vi "IV_Fast.vi"(8 "error in":errorcluster, 11 "Transport":refnum<class "Transport.lvclass">) -> (0 "error out":errorcluster, 3 "Transport out":refnum<class "Transport.lvclass">)   [LabVIEW 2016, in "Transport.lvclass"]
uses:
  Transport.lvclass
  Control Experiment/Typedefs/Instruments--cluster.ctl
  <userlib>/LevyLab/Krohn Hite 7008/Instrument.KH7008.lvclass
  <userlib>/LevyLab/Lockin-Multichannel/Instrument.Lockin/Instrument.Lockin.lvclass
  <userlib>/LevyLab/Levylab Instruments/Instrument Types/Cryostat/Instrument.Cryostat.lvclass
  <userlib>/LevyLab/Levylab Instruments/Instrument Types/CBridge/Instrument.CBridge.lvclass
  <userlib>/LevyLab/Levylab Instruments/Instrument Types/Optical Delay Line/Instrument.OpticalDelayLine.lvclass
  <userlib>/LevyLab/Levylab Instruments/Instrument Types/Strain/Instrument.Strain.lvclass
  <userlib>/LevyLab/Levylab Instruments/Instrument Types/VNA/Instrument.VNA.lvclass
  <userlib>/LevyLab/Levylab Instruments/Instrument Types/VSource/Instrument.VSource.lvclass
  <userlib>/LevyLab/Lockin-Multichannel/LockinDAQ/Typedefs/AO-cluster.ctl
  <userlib>/LevyLab/Lockin-Multichannel/LockinDAQ/Typedefs/Function-enum.ctl
  Transport.lvclass/Transport.ctl
  Control Experiment/Control Experiment.lvclass/Control Experiment.ctl
  Control Experiment/Control Experiment.lvclass
  <userlib>/LevyLab/Lockin-Multichannel/LockinDAQ/LockinDAQ.lvclass
panel:
  in  "OK":bool
  out "4Term":cluster{dbl[], dbl[]}[](graph)
  out "2Term":T1(graph)
  in  "Tab Control":T2(tab)
  in  "decimating factor":i32=1
  in  "low cutoff freq: fl":dbl=0.01 format="%0.4f"
  out "Temp":dbl
  in  "offset":dbl[](array[numeric])=[0.0, 0.0, 0.0, 0.0, 0.0, 0.0, 0.0, 0.0] format="%_6p"
  in  "invert":dbl[](array[numeric])=[1.0, 1.0, 1.0, 1.0, 1.0, 1.0, 1.0, 1.0] format="%#_6p"
  out "DC Voltages":dbl[](array[numeric])=[0.00025, 0.3, 0.0, 0.0, 0.0, 0.0, 0.0, 0.0, 0.00025, 0.3, 0.0, 0.0, 0.0, 0.0, 0.0, 0.0, 0.00025, 0.3, 0.0, 0.0, 0.0, 0.0, 0.0, 0.0, 0.00025, 0.3, 0.0, 0.0, 0.0, 0.0, 0.0, 0.0, 0.00025, 0.3, 0.0, 0.0, 0.0, 0.0, 0.0, 0.0, 0.00025, 0.3, 0.0, 0.0, 0.0, 0.0, 0.0, 0.0, 0.00025, 0.3, 0.0, 0.0, 0.0, 0.0, 0.0, 0.0, 0.00025, 0.3, 0.0, 0.0, 0.0, 0.0, 0.0, 0.0]
  out "Field (T)":dbl
  in  "Enable Filter?":bool
  in  "Experiment Folder":string="6H_IVcurves"
  in  "Experiment Comments":string="SA03036H\nsweep Vsg:-150mV to 600mV, 1mV steps\nB: 7T to -7T\nVbg = -3.9V\nT: 50mK\n\nlockin\n\nI+/-: 2/3 3mV ac+ 250uV dc bias, 0.4 Hz\nV1+/-: 8/4\nV2+/- 6/28\nV3+/V3-: 27/8\nVsg: 1\nVbg :26\n\ntc 300ms order 2"
  out "AI Waveform":waveform(dbl)[](graph)
  out "AO Waveform":waveform(dbl)[](graph)
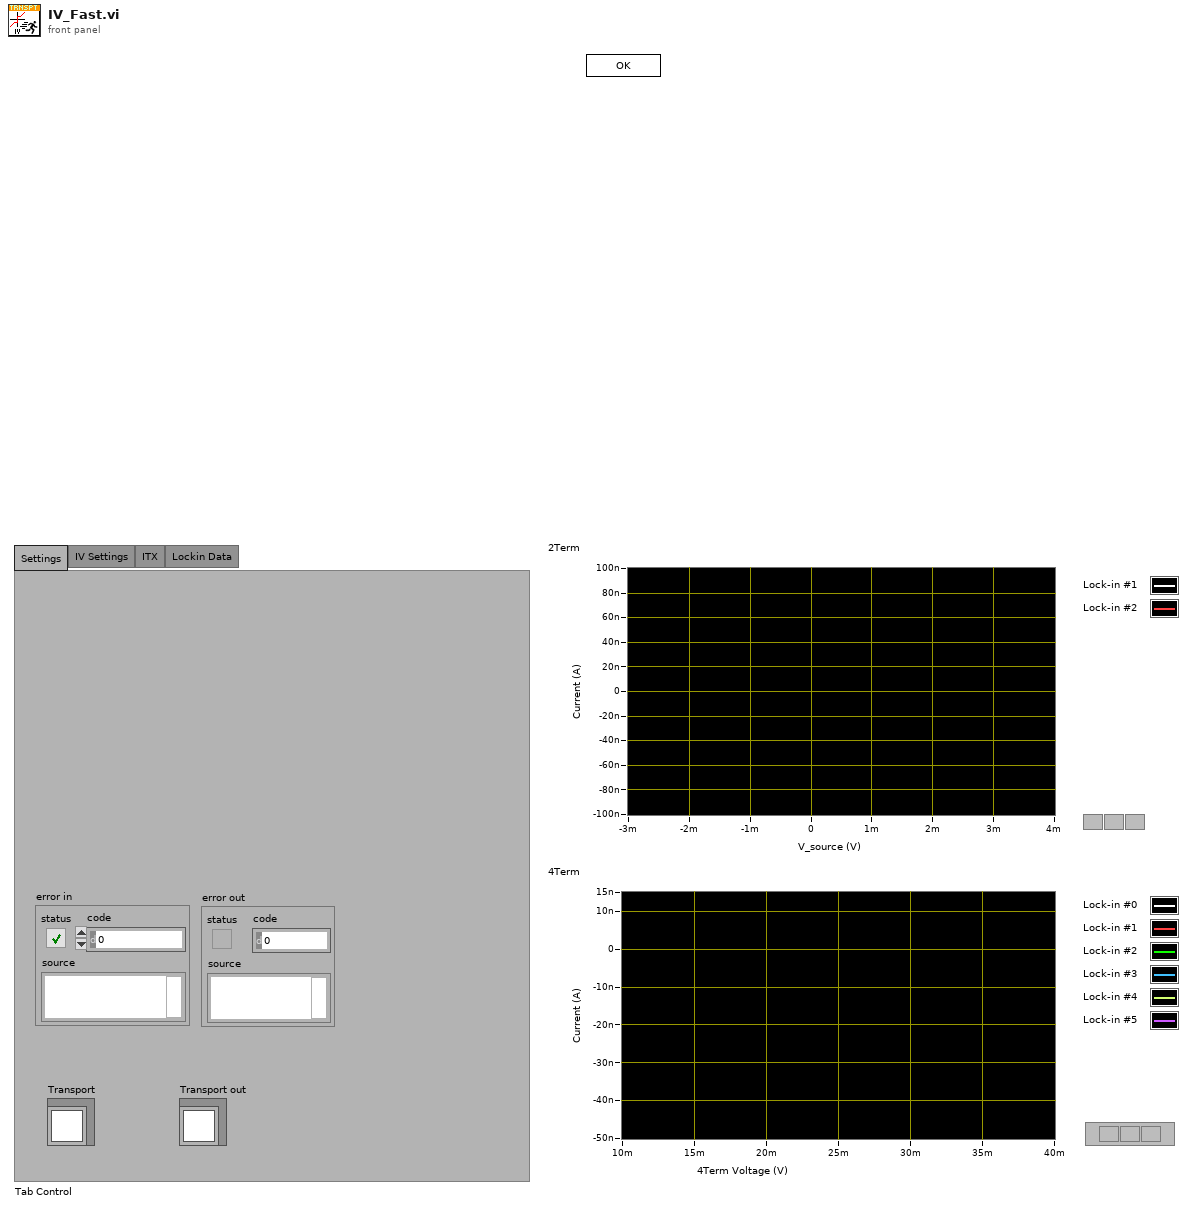
[diagram p1: front panel]
types:
  T1 = cluster{"Decimated and Filtered Array":dbl[], "Decimated and Filtered Array":dbl[]}[]
  T2 = enum32{"Settings", "IV Settings", "ITX", "Lockin Data"}
  T3 = enum32{"Invalid", "Standard", "Closed", "Hidden", "Minimized", "Maximized"}
  T4 = enum32{"invalid app kind", "Development System", "Run Time System", "Student Edition", "Embedded LabVIEW", "Evaluation", "Custom"}
  T5 = typedef "Control Experiment.lvclass/Instruments--cluster.ctl" = cluster{"KH7008":refnum<class "Instrument.KH7008.lvclass">[], "Lockin":refnum<class "Instrument.Lockin.lvclass">, "Temperature":refnum<class "Instrument.Cryostat.lvclass">, "Magnet":refnum<class "Instrument.Cryostat.lvclass">, "Rotator":refnum<class "Instrument.Cryostat.lvclass">, "Level":refnum<class "Instrument.Cryostat.lvclass">, "Capacitance Bridge":refnum<class "Instrument.CBridge.lvclass">, "Optical Delay Line":refnum<class "Instrument.OpticalDelayLine.lvclass">, "Strain Cell":refnum<class "Instrument.Strain.lvclass">, "VNA":refnum<class "Instrument.VNA.lvclass">, "Voltage Source":refnum<class "Instrument.VSource.lvclass">}
  T6 = typedef "LockinDAQ.lvclass/AO-cluster.ctl" = cluster{"Ch":i32[], "Amp (V)":dbl[], "DC (V)":dbl[], "f (Hz)":dbl[], "Phase (°)":dbl[], "Function":T7[], "Sweep?":bool[]}
  T7 = typedef "LockinDAQ.lvclass/Function-enum.ctl" = enum16{"Sine", "Triangle", "Square", "Sawtooth"}
  T8 = cluster{"Core":cluster{"Current VI Reference":refnum<vi>, "Close Panel on Exit?":bool}, "Transport":refnum<class "Transport.lvclass">, "SweepControl":refnum<class "SweepControl.lvclass">, "Control Experiment":refnum<class "Control Experiment.lvclass">, "Instruments":T5, "Temperature":dbl, "Magnet":dbl, "AOconfig":T6, "AO Waveforrm":waveform(dbl)[], "AI Waveform":waveform(dbl)[], "time":dbl[], "time (filtered)":dbl[], "AI (filtered)":cluster{"Decimated and Filtered Array":dbl[]}[], "AO (filtered)":cluster{"Decimated and Filtered Array":dbl[]}[]}
  T9 = cluster{"Current VI Reference":refnum<vi>, "Close Panel on Exit?":bool}
  T10 = enum32{"Bad", "Idle", "Run top level", "Running"}
  T11 = cluster{"I-":i32, "I+":i32, "V1-":i32, "V1+":i32, "I2-":i32, "I2+":i32, "V2-":i32, "V2+":i32}
  T12 = cluster{"Decimated and Filtered Array":dbl[], "Decimated and Filtered Array":dbl[]}
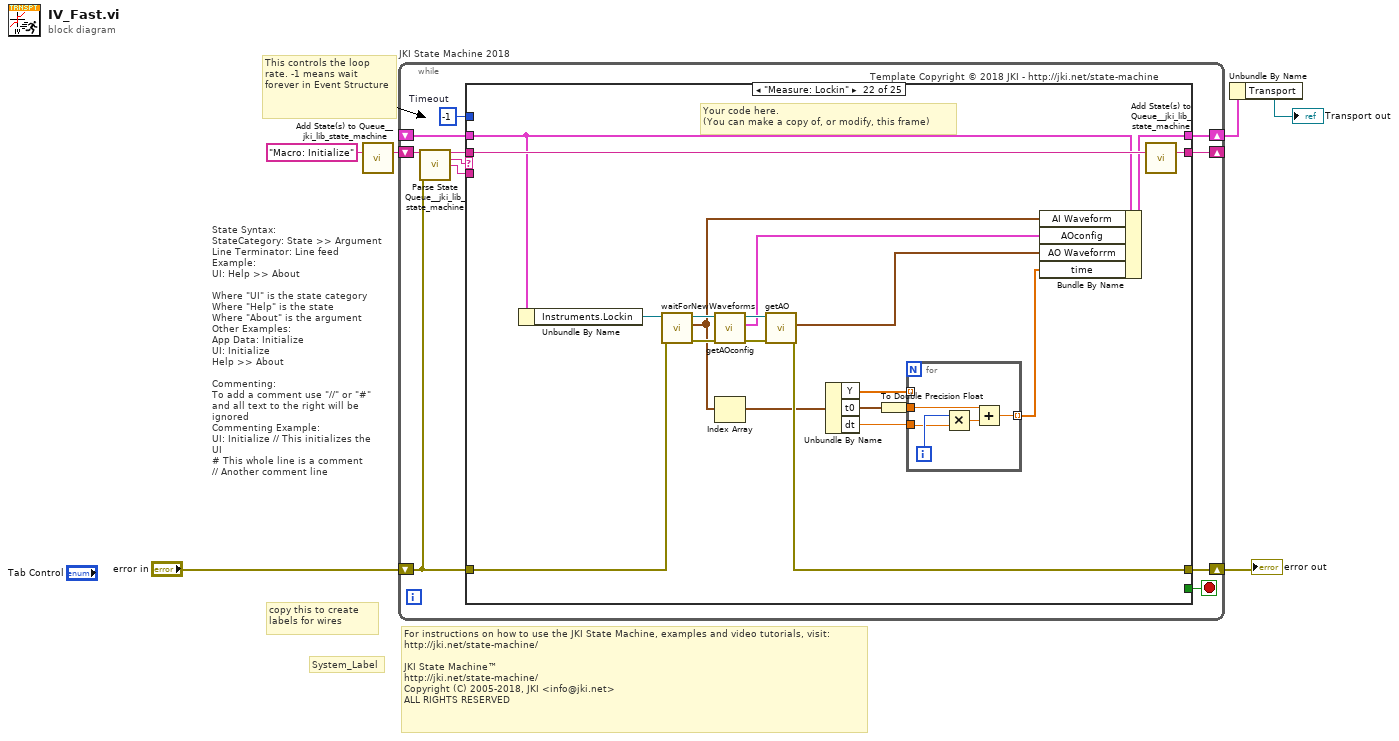
[diagram p0: block diagram]
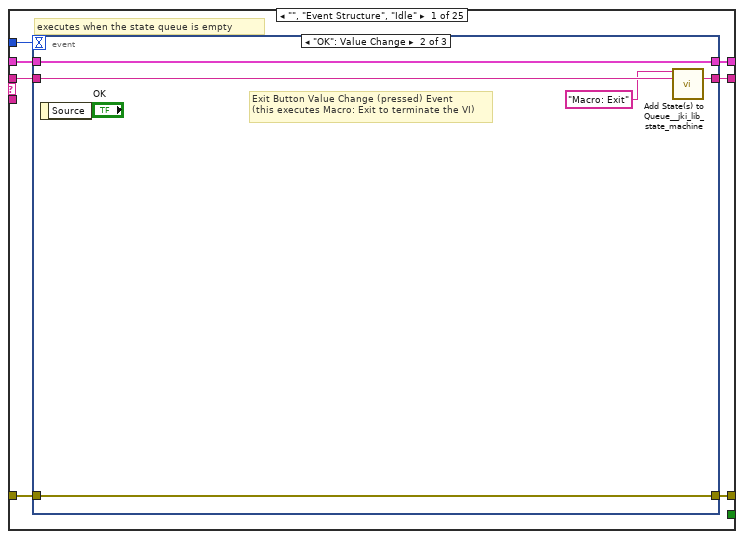
[diagram p2: hidden frame]
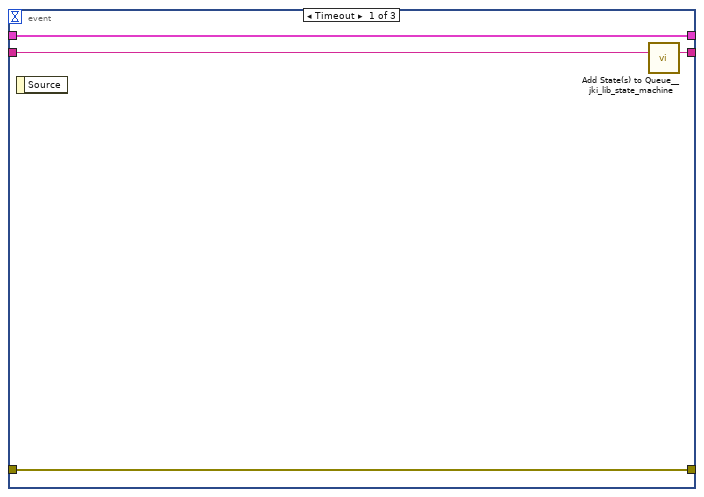
[diagram p3: hidden frame]
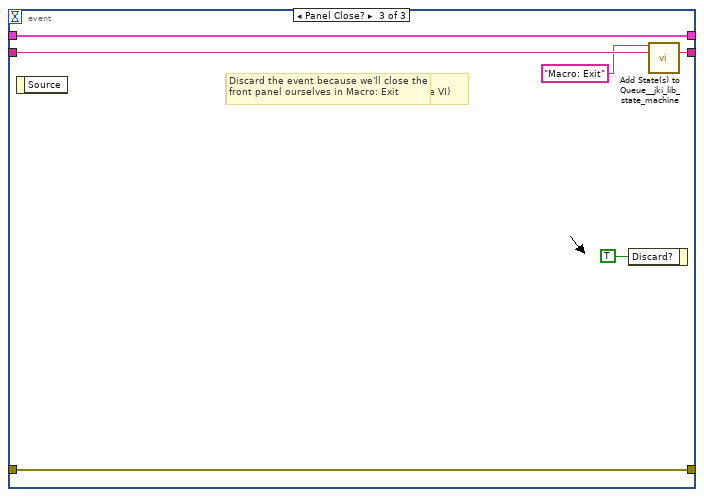
[diagram p4: hidden frame]
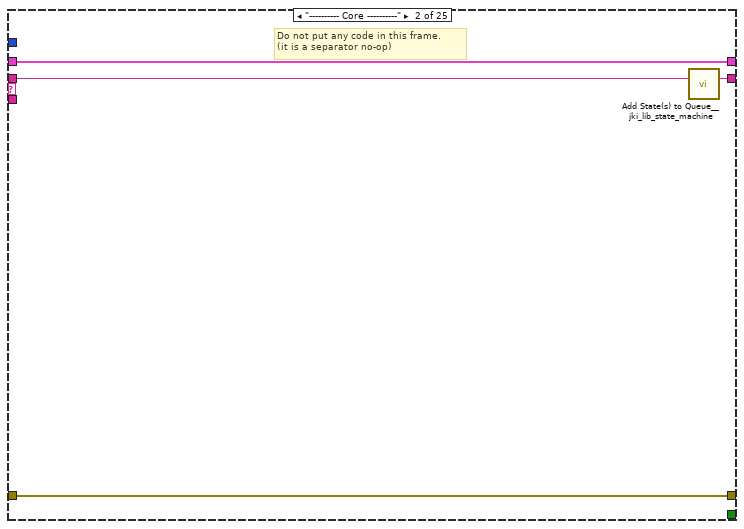
[diagram p5: hidden frame]
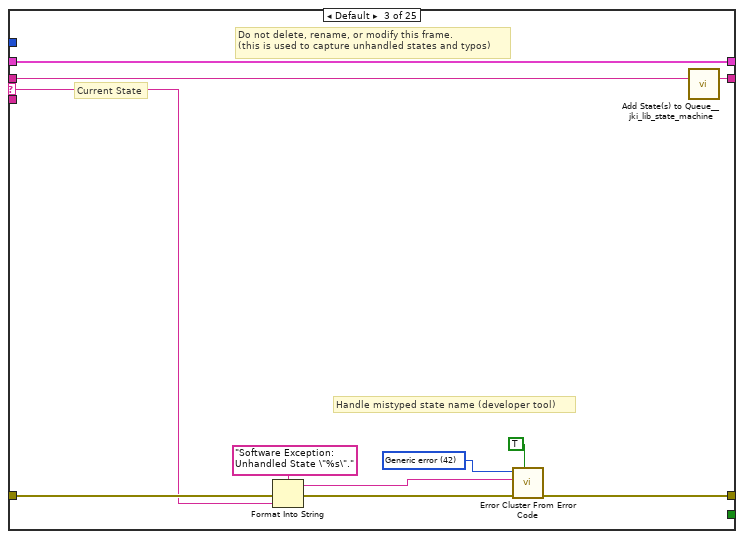
[diagram p6: hidden frame]
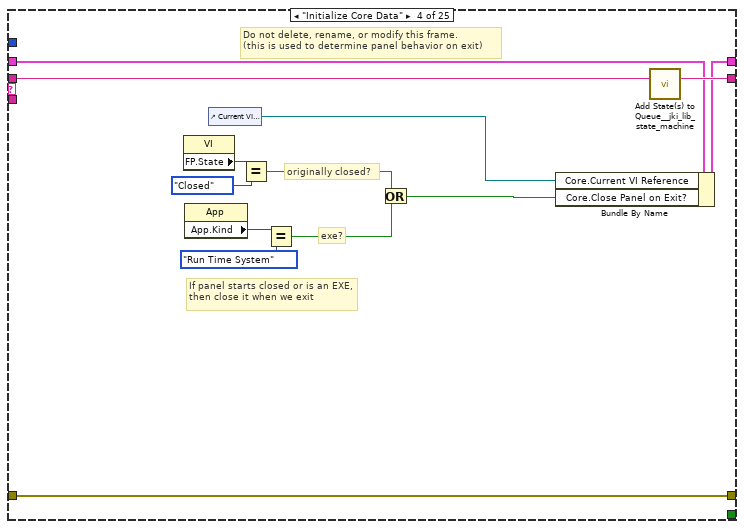
[diagram p7: hidden frame]
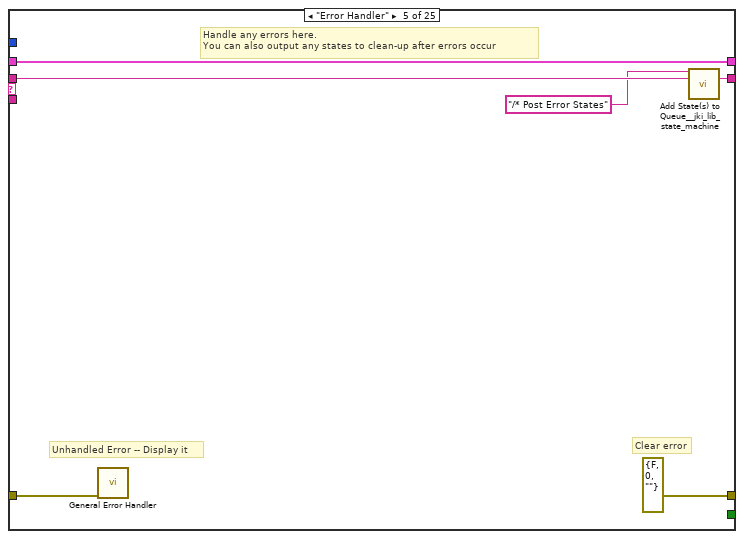
[diagram p8: hidden frame]
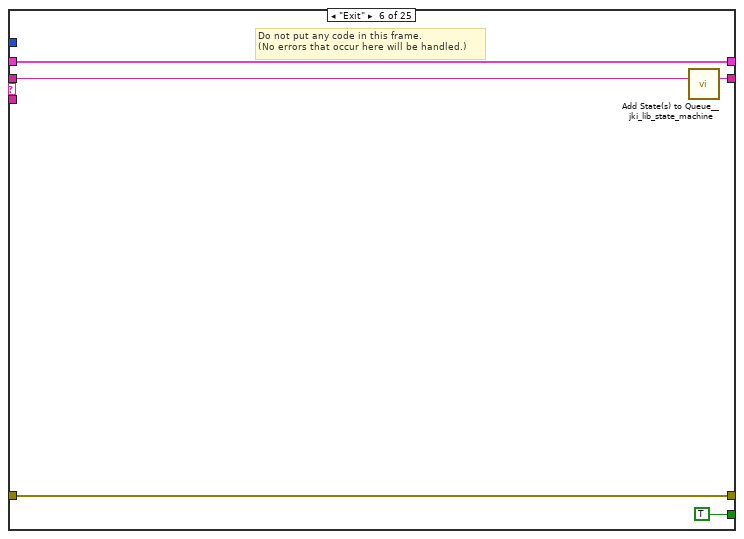
[diagram p9: hidden frame]
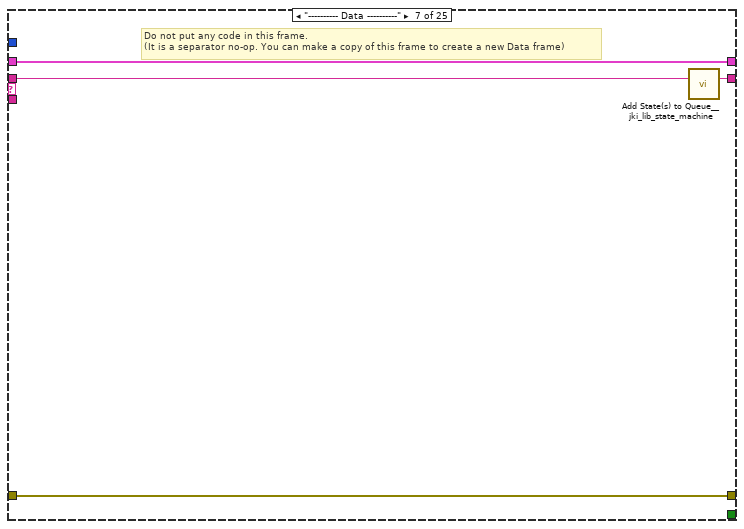
[diagram p10: hidden frame]
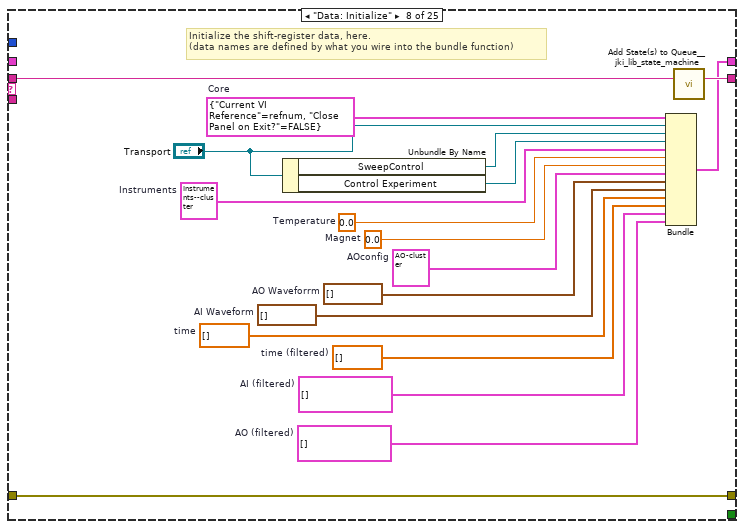
[diagram p11: hidden frame]
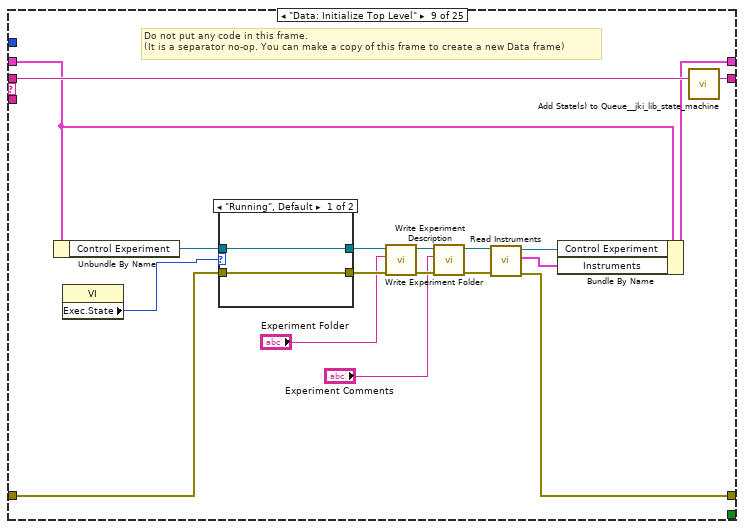
[diagram p12: hidden frame]
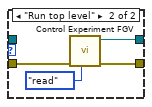
[diagram p13: hidden frame]
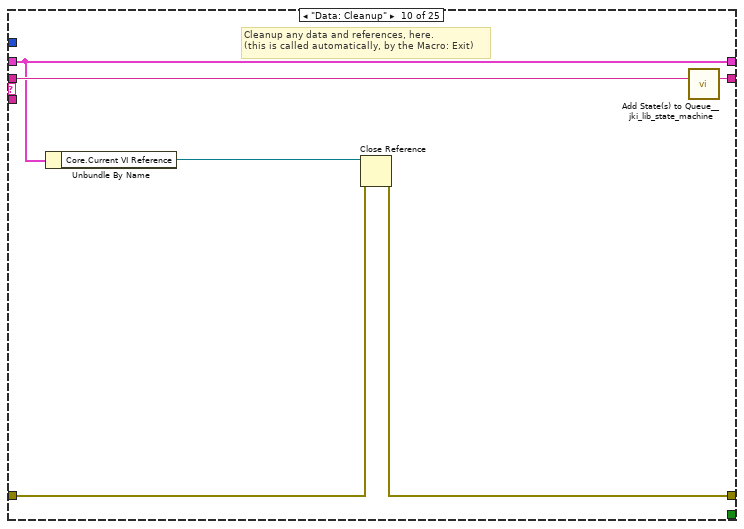
[diagram p14: hidden frame]
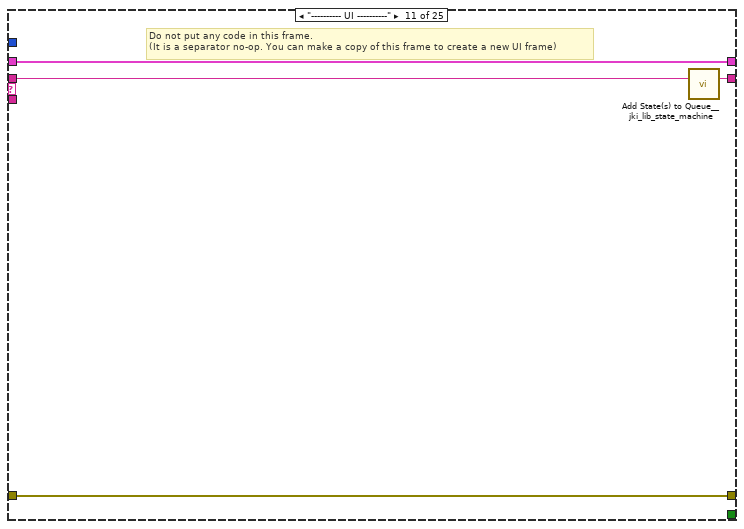
[diagram p15: hidden frame]
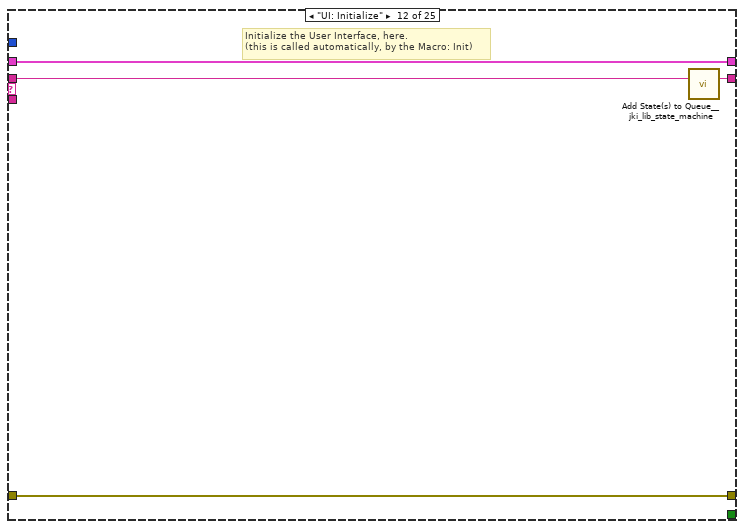
[diagram p16: hidden frame]
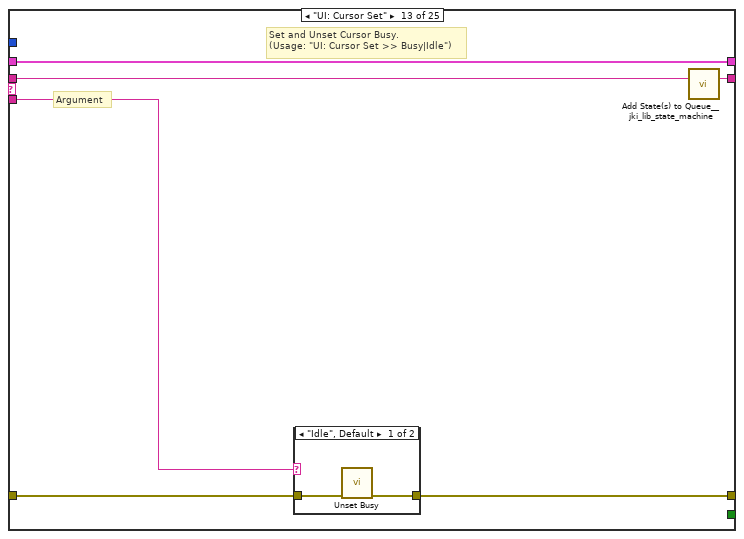
[diagram p17: hidden frame]
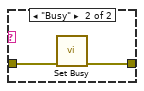
[diagram p18: hidden frame]
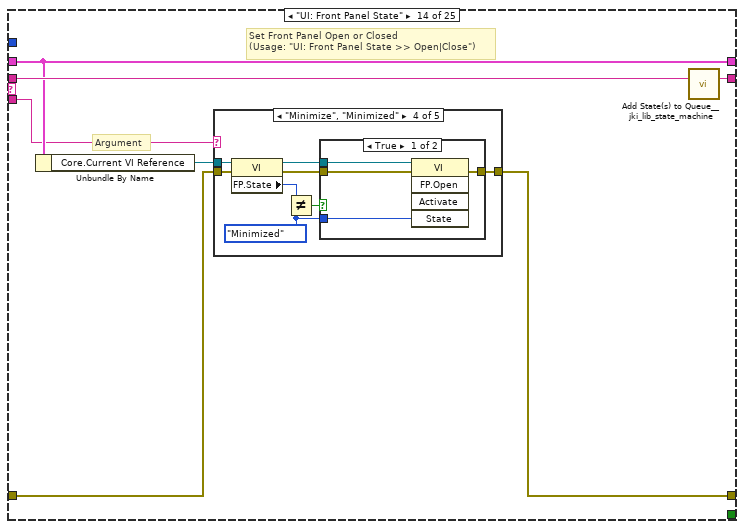
[diagram p19: hidden frame]
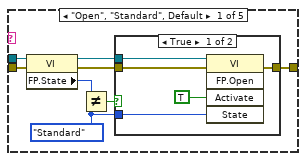
[diagram p20: hidden frame]
diagram:
  # "For instructions on how to use the JKI State Machine, examples and video tutorials, visit:\nhttp://jki.net/state-machine/\n\nJKI State Machine™\nhttp://jki.net/state-machine/\nCopyright (C) 2005-2018, JKI <info@jki.net>\nALL RIGHTS RESERVED"
  # "State Syntax:\nStateCategory: State >> Argument\nLine Terminator: Line feed\nExample:\nUI: Help >> About\n\nWhere \"UI\" is the state category\nWhere \"Help\" is the state\nWhere \"About\" is the argument\nOther Examples:\nApp Data: Initialize\nUI: Initialize\nHelp >> About\n\nCommenting:\nTo add a comment use \"//\" or \"#\" and all text to the right will be ignored\nCommenting Example:\nUI: Initialize // This initializes the UI\n# This whole line is a comment\n// Another comment line"
  # "copy this to create labels for wires"
  # "This controls the loop rate. -1 means wait forever in Event Structure"
  # "System_Label"
  n1 = call <vilib>:"Add State(s) to Queue__jki_lib_state_machine.vi"("State(s) in (\"\")"="Macro: Initialize") -> ("States Out"=w6:string)  [unwired: 14 in]
  n2 = while "JKI State Machine 2018" {
    shift-right: [w10] -> w4
    shift-left: _ -> [w9]
    shift-right: [w13] -> w1
    shift-left: "error in" -> [w7]
    shift-right: [w12] -> _
    shift-left: w6 -> [w14]
    stop <- w11 stop-if-true
    w8 = -1  # Timeout
    # "Template Copyright © 2018 JKI - http://jki.net/state-machine"
    n3 = call <vilib>:"Parse State Queue__jki_lib_state_machine.vi"("State Queue"=w14, "Error In (no error)"=w7) -> ("Remaining States"=w16:string, "Current State"=w17:string, "Arguments"=w15:string)  [unwired: 11 in]
    n4 = case shown="\"Measure: Lockin\"" w17 {
      selector: w17 -> [_ _ w44 _ _ _ _ _ _ _ _ _ _ _ _ _ _ _ _ _ _ _ _ _ _]
      tunnel: w16 -> [w24 w43 w48 w67 w73 w78 w82 w100 w118 w130 w134 w138 w144 w155 w227 w258 w262 w267 w277 w281 w294 w314 w336 w357 w376]
      tunnel: w15 -> [_ _ _ _ _ _ _ _ _ _ _ _ w139 w149 _ _ _ _ _ _ _ _ _ _ _]
      tunnel: w9 -> [w22 w40 w46 w60 w70 w76 w79 _ w102 w125 w131 w136 w142 w151 w221 w238 w259 w264 w274 w278 w286 w298 w323 w354 w371]
      tunnel: [w21 w41 w50 w64 errorcluster {"status"=FALSE, "code"=0, "source"=""} ("error out") w75 w80 w97 w106 w126 w132 w135 w140 w152 w225 w231 w260 w265 w275 w279 w283 w307 w334 w355 w358] -> w13
      tunnel: w7 -> [w20 w41 w49 w64 w69 w75 w80 w97 w107 w127 w132 w135 w141 w153 w225 w232 w260 w265 w275 w279 w289 w308 w334 w355 w359]
      tunnel: [w23 w42 w47 w66 w72 w77 w81 w99 w117 w129 w133 w137 w143 w154 w226 w257 w261 w266 w276 w280 w293 w313 w335 w356 w375] -> w12
      tunnel: [_ _ _ _ _ TRUE _ _ _ _ _ _ _ _ _ _ _ _ _ _ _ _ _ _ _] -> w11
      tunnel: [w19 w40 w46 w65 w70 w76 w79 w98 w101 w125 w131 w136 w142 w151 w221 w238 w259 w264 w274 w278 w285 w297 w322 w354 w371] -> w10
      tunnel: w8 -> [w18 _ _ _ _ _ _ _ _ _ _ _ _ _ _ _ _ _ _ _ _ _ _ _ _]
      frame "", "Event Structure", "Idle" {
        # "executes when the state queue is empty"
        n5 = event shown="[1] \"OK\": Value Change" {
          selector: _ -> [_ _ _]
          dyn-events: _ -> [_ _ _]
          timeout: w18 -> [_ _ _]
          tunnel: w24 -> [w28 w33 w39]
          tunnel: [w27 w32 w38] -> w23
          tunnel: w22 -> [w25 w30 w36]
          tunnel: [w26 w31 w37] -> w21
          tunnel: w20 -> [w26 w31 w37]
          tunnel: [w25 w30 w36] -> w19
          event Timeout {
            n6 = event-data() -> ()  [unwired: 1 in, 1 out]
            n7 = call <vilib>:"Add State(s) to Queue__jki_lib_state_machine.vi"("State(s) in (\"\")"=w28) -> ("States Out"=w27:string)  [unwired: 14 in]
          }
          event "OK": Value Change {
            # "Exit Button Value Change (pressed) Event\n(this executes Macro: Exit to terminate the VI)"
            n8 = event-data() -> ()  [unwired: 1 in, 1 out]
            n9 = call <vilib>:"Add State(s) to Queue__jki_lib_state_machine.vi"("State(s) in Front (\"\")"="Macro: Exit", "State(s) in (\"\")"=w33) -> ("States Out"=w32:string)  [unwired: 13 in]
          }
          event Panel Close? {
            # "Discard the event because we'll close the front panel ourselves in Macro: Exit"
            # "Close Panel button (pressed) Event\n(this executes Macro: Exit to terminate the VI)"
            n10 = event-data() -> ()  [unwired: 1 in, 1 out]
            n11 = event-data("Discard?"=TRUE) -> ()  [unwired: 1 in, 1 out]
            n12 = call <vilib>:"Add State(s) to Queue__jki_lib_state_machine.vi"("State(s) in Front (\"\")"="Macro: Exit", "State(s) in (\"\")"=w39) -> ("States Out"=w38:string)  [unwired: 13 in]
          }
        }
      }
      frame "---------- Core ----------" {
        # "Do not put any code in this frame.\n(it is a separator no-op)"
        n13 = call <vilib>:"Add State(s) to Queue__jki_lib_state_machine.vi"("State(s) in (\"\")"=w43) -> ("States Out"=w42:string)  [unwired: 14 in]
      }
      frame Default {
        w53 = 42 items=["No error", "Argument error", "Memory is full", "Out of zone", "End of file", "File already open", "Generic file I/O error", "File not found", "File permission error", "Disk is full", "Duplicate path", "Too many files open", "System feature not enabled", "Resource file not found", "Cannot add resource", "Resource not found", "Image not found", "Image memory error", "Pen does not exist", "Config type invalid", "Config token not found", "Config parse error", "Config memory error", "Bad external code format", "Bad external code offset", "External code not present", "Null window", "Destroy window error", "Null menu", "Print aborted", "Bad print record", "Print driver error", "Windows error during printing", "Memory error during printing", "Print dialog error", "Generic print error", "Invalid device refnum", "Device not found", "Device parameter error", "Device unit error", "Cannot open device", "Device call aborted", "Generic error", "Cancelled by user", "Object ID too low", "Object ID too high", "Object not in heap", "Unknown heap", "Unknown object (invalid DefProc)", "Unknown object (DefProc not in table)", "Message out of range", "Invalid (null) method", "Unknown message", "Manager call not supported", "Bad address", "Network operation in progress", "Network operation timed out", "Connection is busy", "Network attribute not supported", "Network error", "Address in use", "System out of memory", "Connection aborted", "Connection refused", "Not connected", "Already connected", "Connection closed", "Initialization error (interapplication manager)", "Bad occurrence", "Wait on unbound occurrence handler", "Occurrence queue overflow", "Datalog type conflict", "Unused", "Unrecognized type (interapplication manager)", "Memory corrupt", "Failed to make temporary DLL", "Old CIN version", "Drag socket not found", "Failed to load drop-object", "Failed to register OLE object", "Failed to release OLE object", "Format specifier type mismatch", "Unknown format specifier", "Too few format specifiers", "Too many format specifiers", "Scan failed", "Newer CIN version", "Error converting to variant", "Runtime menu error", "Password tampered", "Variant attribute not found", "Incompatible variant data type", "Event data is not available", "Event Store is not present", "Occurrence is not found", "Event Queue is not created", "Event info is not available", "Refnum passed is NULL", "Error retrieving Class GUID", "Error retrieving CoClass GUID", "Error retrieving TypeLib GUID.", "Bad built application magic bytes.", "Specific driver is different from the specific driver associated with the Logical Name.", "There is no session opened to the class driver.", "Max Error", "MAX - Error with config objects", "MAX - Error loading configuration", "MAX - Group not supported"]
        # "Current State"
        # "Do not delete, rename, or modify this frame.\n(this is used to capture unhandled states and typos)"
        # "Handle mistyped state name (developer tool)"
        n14 = Format Into String(format string="Software Exception: Unhandled State \"%s\"." ("message"), error in=w49, w44) -> (resulting string=w52:string, error out=w51:errorcluster)  [unwired: 1 in]
        n15 = call <vilib>:"Error Cluster From Error Code.vi"("show call chain? (False)"=TRUE, "error in (no error)"=w51, "error message (\"\")"=w52, "error code (0)"=w53) -> ("error out"=w50:errorcluster)  [unwired: 5 in]
        n16 = call <vilib>:"Add State(s) to Queue__jki_lib_state_machine.vi"("State(s) in (\"\")"=w48) -> ("States Out"=w47:string)  [unwired: 14 in]
      }
      frame "Initialize Core Data" {
        # "Do not delete, rename, or modify this frame.\n(this is used to determine panel behavior on exit)"
        # "originally closed?"
        # "exe?"
        # "If panel starts closed or is an EXE, then close it when we exit"
        n17 = property class="VI"() -> ("FP.State"=w57:T3)  [unwired: 2 in, 2 out]
        n18 = property class="App"() -> ("App.Kind"=w63:T4)  [unwired: 2 in, 2 out]
        n19 = control-ref of="Current VI Reference"() -> (w58:refnum<vi>)
        n20 = Equal?(x=w57, y=T3."Closed" ("Front Panel Window:State")) -> (x = y?=w55:bool)
        n21 = Equal?(x=w63, y=T4."Run Time System" ("Application:Kind")) -> (x = y?=w61:bool)
        n22 = Or(x=w55, y=w61) -> (x .or. y?=w59:bool)
        n23 = Bundle By Name(cluster=w60, "Core.Current VI Reference"=w58, "Core.Close Panel on Exit?"=w59) -> (w65:T8)
        n24 = call <vilib>:"Add State(s) to Queue__jki_lib_state_machine.vi"("State(s) in (\"\")"=w67) -> ("States Out"=w66:string)  [unwired: 14 in]
      }
      frame "Error Handler" {
        # "Unhandled Error -- Display it"
        # "Handle any errors here.\nYou can also output any states to clean-up after errors occur"
        # "Clear error"
        n25 = call <vilib>:"General Error Handler.vi"("error in (no error)"=w69) -> ()  [unwired: 10 in, 5 out]
        n26 = call <vilib>:"Add State(s) to Queue__jki_lib_state_machine.vi"("State(s) in Front (\"\")"="/* Post Error States", "State(s) in (\"\")"=w73) -> ("States Out"=w72:string)  [unwired: 13 in]
      }
      frame "Exit" {
        # "Do not put any code in this frame.\n(No errors that occur here will be handled.)"
        n27 = call <vilib>:"Add State(s) to Queue__jki_lib_state_machine.vi"("State(s) in (\"\")"=w78) -> ("States Out"=w77:string)  [unwired: 14 in]
      }
      frame "---------- Data ----------" {
        # "Do not put any code in this frame.\n(It is a separator no-op. You can make a copy of this frame to create a new Data frame)"
        n28 = call <vilib>:"Add State(s) to Queue__jki_lib_state_machine.vi"("State(s) in (\"\")"=w82) -> ("States Out"=w81:string)  [unwired: 14 in]
      }
      frame "Data: Initialize" {
        w83 = 0.0  # Magnet
        w84 = 0.0  # Temperature
        w85 = cluster{"Decimated and Filtered Array":dbl[]}[] []  # AO (filtered)
        w86 = cluster{"Decimated and Filtered Array":dbl[]}[] []  # AI (filtered)
        w87 = dbl[] []  # time (filtered)
        w88 = dbl[] []  # time
        w90 = waveform(dbl)[] []  # AO Waveforrm
        w91 = T6 {"Ch"=[], "Amp (V)"=[0.01, 0.0, 0.0, 0.0, 0.0, 0.0, 0.0, 0.0], "DC (V)"=[0.0, 0.0, 0.0, 0.0, 0.0, 0.0, 0.0, 0.0], "f (Hz)"=[0.0, 0.0, 0.0, 0.0, 0.0, 0.0, 0.0, 0.0], "Phase (°)"=[13.1, 13.0, 13.0, 13.0, 13.0, 13.0, 13.0, 13.0], "Function"=[enum."Sine", enum."Sine", enum."Sine", enum."Sine", enum."Sine", enum."Sine", enum."Sine", enum."Sine"], "Sweep?"=[]}  # AOconfig
        w89 = waveform(dbl)[] []  # AI Waveform
        w92 = T5 {"KH7008"=[], "Lockin"=refnum, "Temperature"=refnum, "Magnet"=refnum, "Rotator"=refnum, "Level"=refnum, "Capacitance Bridge"=refnum, "Optical Delay Line"=refnum, "Strain Cell"=refnum, "VNA"=refnum, "Voltage Source"=refnum}  # Instruments
        w96 = T9 {"Current VI Reference"=refnum, "Close Panel on Exit?"=FALSE}  # Core
        # "Initialize the shift-register data, here.\n(data names are defined by what you wire into the bundle function)"
        n29 = Unbundle By Name("Transport") -> ("SweepControl"=w94:refnum<class "SweepControl.lvclass">, "Control Experiment"=w93:refnum<class "Control Experiment.lvclass">)
        n30 = Bundle("Core"=w96, "Transport"="Transport", "SweepControl"=w94, "Control Experiment"=w93, "Instruments"=w92, "Temperature"=w84, "Magnet"=w83, "AOconfig"=w91, "AO Waveforrm"=w90, "AI Waveform"=w89, "time"=w88, "time (filtered)"=w87, "AI (filtered)"=w86, "AO (filtered)"=w85) -> (w98:T8)  [unwired: 1 in]
        n31 = call <vilib>:"Add State(s) to Queue__jki_lib_state_machine.vi"("State(s) in (\"\")"=w100) -> ("States Out"=w99:string)  [unwired: 14 in]
      }
      frame "Data: Initialize Top Level" {
        # "Do not put any code in this frame.\n(It is a separator no-op. You can make a copy of this frame to create a new Data frame)"
        n32 = Unbundle By Name(w102) -> ("Control Experiment"=w110:refnum<class "Control Experiment.lvclass">)
        n33 = property class="VI"() -> ("Exec.State"=w103:T10)  [unwired: 2 in, 2 out]
        n34 = case shown="\"Running\", Default" w103 {
          tunnel: [w120 w124] -> w114
          tunnel: [w119 w123] -> w113
          tunnel: w110 -> [w120 _]
          tunnel: w107 -> [w119 w122]
          frame "Running", Default {
          }
          frame "Run top level" {
            n35 = call "Control Experiment FGV.vi"("Function"=enum16{"read", "write"}."read", "error in (no error)"=w122) -> ("error out"=w123:errorcluster, "Control Experiment.lvclass out"=w124:refnum<class "Control Experiment.lvclass">)  [unwired: 8 in]
          }
        }
        n36 = call "Write Experiment Folder.vi"("error in (no error)"=w113, "Experiment Folder"="Experiment Folder", "Control Experiment in"=w114) -> ("error out"=w111:errorcluster, "Control Experiment out"=w112:refnum<class "Control Experiment.lvclass">)  [unwired: 7 in]
        n37 = call "Write Experiment Description.vi"("error in (no error)"=w111, "Experiment Description"="Experiment Comments", "Control Experiment in"=w112) -> ("error out"=w109:errorcluster, "Control Experiment out"=w108:refnum<class "Control Experiment.lvclass">)  [unwired: 7 in]
        n38 = call "Read Instruments.vi"("error in (no error)"=w109, "Control Experiment in"=w108) -> ("error out"=w106:errorcluster, "Instruments"=w115:T5, "Control Experiment out"=w116:refnum<class "Control Experiment.lvclass">)  [unwired: 7 in]
        n39 = Bundle By Name(cluster=w102, "Control Experiment"=w116, "Instruments"=w115) -> (w101:T8)
        n40 = call <vilib>:"Add State(s) to Queue__jki_lib_state_machine.vi"("State(s) in (\"\")"=w118) -> ("States Out"=w117:string)  [unwired: 14 in]
      }
      frame "Data: Cleanup" {
        # "Cleanup any data and references, here.\n(this is called automatically, by the Macro: Exit)"
        n41 = Unbundle By Name(w125) -> ("Core.Current VI Reference"=w128:refnum<vi>)
        n42 = Close Reference(reference=w128, error in (no error)=w127) -> (error out=w126:errorcluster)
        n43 = call <vilib>:"Add State(s) to Queue__jki_lib_state_machine.vi"("State(s) in (\"\")"=w130) -> ("States Out"=w129:string)  [unwired: 14 in]
      }
      frame "---------- UI ----------" {
        # "Do not put any code in this frame.\n(It is a separator no-op. You can make a copy of this frame to create a new UI frame)"
        n44 = call <vilib>:"Add State(s) to Queue__jki_lib_state_machine.vi"("State(s) in (\"\")"=w134) -> ("States Out"=w133:string)  [unwired: 14 in]
      }
      frame "UI: Initialize" {
        # "Initialize the User Interface, here.\n(this is called automatically, by the Macro: Init)"
        n45 = call <vilib>:"Add State(s) to Queue__jki_lib_state_machine.vi"("State(s) in (\"\")"=w138) -> ("States Out"=w137:string)  [unwired: 14 in]
      }
      frame "UI: Cursor Set" {
        # "Argument"
        # "Set and Unset Cursor Busy.\n(Usage: \"UI: Cursor Set >> Busy|Idle\")"
        n46 = case shown="\"Idle\", Default" w139 {
          tunnel: w141 -> [w146 w148]
          tunnel: [w145 w147] -> w140
          frame "Idle", Default {
            n47 = call <vilib>:"Unset Busy.vi"("error in (no error)"=w146) -> ("error out"=w145:errorcluster)  [unwired: 10 in]
          }
          frame "Busy" {
            n48 = call <vilib>:"Set Busy.vi"("error in (no error)"=w148) -> ("error out"=w147:errorcluster)  [unwired: 9 in, 1 out]
          }
        }
        n49 = call <vilib>:"Add State(s) to Queue__jki_lib_state_machine.vi"("State(s) in (\"\")"=w144) -> ("States Out"=w143:string)  [unwired: 14 in]
      }
      frame "UI: Front Panel State" {
        # "Argument"
        # "Set Front Panel Open or Closed\n(Usage: \"UI: Front Panel State >> Open|Close\")"
        n50 = Unbundle By Name(w151) -> ("Core.Current VI Reference"=w150:refnum<vi>)
        n51 = case shown="\"Minimize\", \"Minimized\"" w149 {
          tunnel: w153 -> [w161 w176 w187 w200 w213]
          tunnel: [w163 w177 w189 w202 w215] -> w152
          tunnel: w150 -> [w162 w174 w188 w201 w214]
          frame "Open", "Standard", Default {
            w156 = T3."Standard" ("State")
            n52 = property class="VI"(reference=w162, error in=w161) -> (reference out=w159:refnum<vi>, error out=w160:errorcluster, "FP.State"=w158:T3)
            n53 = Not Equal?(x=w158, y=w156) -> (x != y?=w157:bool)
            n54 = case shown="True" w157 {
              tunnel: [w167 w169] -> w163
              tunnel: w160 -> [w166 w169]
              tunnel: w159 -> [w165 _]
              tunnel: w156 -> [w164 _]
              frame True {
                n55 = invoke class="VI" method="FP.Open"(reference=w165, error in=w166, "Activate"=TRUE, "State"=w164) -> (error out=w167:errorcluster)  [unwired: 1 in, 4 out]
              }
              frame False {
              }
            }
          }
          frame "Close", "Closed" {
            n56 = property class="VI"(reference=w174, error in=w176) -> (reference out=w173:refnum<vi>, error out=w175:errorcluster, "FP.State"=w171:T3)
            n57 = Not Equal?(x=w171, y=T3."Closed" ("Front Panel Window:State")) -> (x != y?=w170:bool)
            n58 = case shown="True" w170 {
              tunnel: [w178 w181] -> w177
              tunnel: w175 -> [w178 w180]
              tunnel: w173 -> [_ w179]
              frame False {
              }
              frame True {
                n59 = invoke class="VI" method="FP.Close"(reference=w179, error in=w180) -> (error out=w181:errorcluster)  [unwired: 1 in, 2 out]
              }
            }
          }
          frame "Hidden", "Hide" {
            w182 = T3."Hidden" ("State")
            n60 = property class="VI"(reference=w188, error in=w187) -> (reference out=w185:refnum<vi>, error out=w186:errorcluster, "FP.State"=w184:T3)
            n61 = Not Equal?(x=w184, y=w182) -> (x != y?=w183:bool)
            n62 = case shown="True" w183 {
              tunnel: [w193 w194] -> w189
              tunnel: w186 -> [w192 w194]
              tunnel: w185 -> [w191 _]
              tunnel: w182 -> [w190 _]
              frame True {
                n63 = invoke class="VI" method="FP.Open"(reference=w191, error in=w192, "State"=w190) -> (error out=w193:errorcluster)  [unwired: 2 in, 4 out]
              }
              frame False {
              }
            }
          }
          frame "Minimize", "Minimized" {
            w195 = T3."Minimized" ("State")
            n64 = property class="VI"(reference=w201, error in=w200) -> (reference out=w198:refnum<vi>, error out=w199:errorcluster, "FP.State"=w197:T3)
            n65 = Not Equal?(x=w197, y=w195) -> (x != y?=w196:bool)
            n66 = case shown="True" w196 {
              tunnel: [w206 w207] -> w202
              tunnel: w199 -> [w205 w207]
              tunnel: w198 -> [w204 _]
              tunnel: w195 -> [w203 _]
              frame True {
                n67 = invoke class="VI" method="FP.Open"(reference=w204, error in=w205, "State"=w203) -> (error out=w206:errorcluster)  [unwired: 2 in, 4 out]
              }
              frame False {
              }
            }
          }
          frame "Maximize", "Maximized" {
            w208 = T3."Maximized" ("State")
            n68 = property class="VI"(reference=w214, error in=w213) -> (reference out=w211:refnum<vi>, error out=w212:errorcluster, "FP.State"=w210:T3)
            n69 = Not Equal?(x=w210, y=w208) -> (x != y?=w209:bool)
            n70 = case shown="True" w209 {
              tunnel: [w219 w220] -> w215
              tunnel: w212 -> [w218 w220]
              tunnel: w211 -> [w217 _]
              tunnel: w208 -> [w216 _]
              frame True {
                n71 = invoke class="VI" method="FP.Open"(reference=w217, error in=w218, "State"=w216) -> (error out=w219:errorcluster)  [unwired: 2 in, 4 out]
              }
              frame False {
              }
            }
          }
        }
        n72 = call <vilib>:"Add State(s) to Queue__jki_lib_state_machine.vi"("State(s) in (\"\")"=w155) -> ("States Out"=w154:string)  [unwired: 14 in]
      }
      frame "UI: Update Input Graphs" {
        # "Do not put any code in this frame.\n(It is a separator no-op. You can make a copy of this frame to create a new UI frame)"
        n73 = Unbundle By Name(w221) -> ("AOconfig.DC (V)"=→"DC Voltages":dbl[], "AO Waveforrm"=→"AO Waveform":waveform(dbl)[], "AI Waveform"=→"AI Waveform":waveform(dbl)[])
        n74 = call <vilib>:"Add State(s) to Queue__jki_lib_state_machine.vi"("State(s) in (\"\")"=w227) -> ("States Out"=w226:string)  [unwired: 14 in]
      }
      frame "UI: Update IV Graphs" {
        # "Decimated AO"
        # "Decimataed AI"
        # "Do not put any code in this frame.\n(It is a separator no-op. You can make a copy of this frame to create a new UI frame)"
        n75 = Unbundle By Name(w238) -> ("AI (filtered)"=w237:cluster{"Decimated and Filtered Array":dbl[]}[], "AO (filtered)"=w236:cluster{"Decimated and Filtered Array":dbl[]}[], "Control Experiment"=w233:refnum<class "Control Experiment.lvclass">)
        n76 = call "Get Channel Indices.vi"("error in (no error)"=w232, "Control Experiment in"=w233) -> ("error out"=w231:errorcluster, "Indices"=w228:T11)  [unwired: 7 in, 1 out]
        n77 = Unbundle By Name(w228) -> ("I-"=w235:i32, "V1+"=w229:i32, "V1-"=w230:i32, "I+"=w234:i32)
        n78 = Decrement(x=w235) -> (x-1=w241:i32)
        n79 = Decrement(x=w229) -> (x-1=w250:i32)
        n80 = Decrement(x=w230) -> (x-1=w244:i32)
        n81 = Decrement(x=w234) -> (x-1=w253:i32)
        n82 = Index Array(array=w236, index=w253) -> (element=w254:cluster{"Decimated and Filtered Array":dbl[]})
        n83 = Index Array(array=w237, index #1=w241, index #2=w250, index #3=w244) -> (element #1=w247:cluster{"Decimated and Filtered Array":dbl[]}, element #2=w243:cluster{"Decimated and Filtered Array":dbl[]}, element #3=w249:cluster{"Decimated and Filtered Array":dbl[]})
        n84 = Equal?(x=w250, y=w244) -> (x = y?=w245:bool)
        n85 = Subtract(x=w243, y=w249) -> (x-y=w242:cluster{"Decimated and Filtered Array":dbl[]})
        n86 = Select(t=w243, s=w245, f=w242) -> (s? t:f=w246:cluster{"Decimated and Filtered Array":dbl[]})
        n87 = Unbundle(w247) -> ("Decimated and Filtered Array"=w251:dbl[])
        n88 = Unbundle(w254) -> ("Decimated and Filtered Array"=w252:dbl[])
        n89 = Unbundle(w246) -> ("Decimated and Filtered Array"=w248:dbl[])
        n90 = Bundle("Decimated and Filtered Array"=w248, "Decimated and Filtered Array"=w251) -> (w239:T12)  [unwired: 1 in]
        n91 = Bundle("Decimated and Filtered Array"=w252, "Decimated and Filtered Array"=w251) -> (w255:T12)  [unwired: 1 in]
        n92 = Build Array(w239) -> (→"4Term":T1)
        n93 = Build Array(w255) -> (→"2Term":T1)
        n94 = call <vilib>:"Add State(s) to Queue__jki_lib_state_machine.vi"("State(s) in (\"\")"=w258) -> ("States Out"=w257:string)  [unwired: 14 in]
      }
      frame "---------- Macro ----------" {
        # "Do not put any code in this frame.\n(It is a separator no-op. You can make a copy of this frame to create a new Macro frame)"
        n95 = call <vilib>:"Add State(s) to Queue__jki_lib_state_machine.vi"("State(s) in (\"\")"=w262) -> ("States Out"=w261:string)  [unwired: 14 in]
      }
      frame "Macro: Initialize" {
        w263 = "Data: Initialize\nInitialize Core Data\nUI: Initialize\nUI: Front Panel State >> Open\nData: Initialize Top Level\nMeasure: Cryostat\nMeasure: Lockin\nMeasure: Filter and Decimate\nUI: Update Input Graphs\nUI: Update IV Graphs\nFile: Save\nMacro: Exit"  # Data: Initialize Initialize Core Data UI: Initialize UI: Front Panel State >> Open Data: Initialize Top Level Measure: Cryostat Measure: Lockin Measure: Filter and Decimate UI: Update Input Graphs UI: Update IV Graphs File: Save Macro: Exit
        # "Initialization Macro\n(This is called once, when the VI starts)"
        n96 = call <vilib>:"Add State(s) to Queue__jki_lib_state_machine.vi"("State(s) in Front (\"\")"=w263, "State(s) in (\"\")"=w267) -> ("States Out"=w266:string)  [unwired: 13 in]
      }
      frame "Macro: Exit" {
        # "Exit Macro\n(This is called once, when the VI exits)"
        n97 = Unbundle By Name(w274) -> ("Core.Close Panel on Exit?"=w273:bool)
        n98 = Select(t="UI: Front Panel State >> Close", s=w273, f="") -> (s? t:f=w270:string)
        n99 = call <vilib>:"Add State(s) to Queue__jki_lib_state_machine.vi"("State(s) in (\"\")"=w270, "State(s) at Back (\"\")"="Data: Cleanup\nExit") -> ("States Out"=w268:string)  [unwired: 13 in]
        n100 = call <vilib>:"Add State(s) to Queue__jki_lib_state_machine.vi"("State(s) in Front (\"\")"=w268, "State(s) in (\"\")"=w277) -> ("States Out"=w276:string)  [unwired: 13 in]
      }
      frame "---------- Measure ----------" {
        # "Template Separator\n(You can make a copy of, or modify, this frame)"
        n101 = call <vilib>:"Add State(s) to Queue__jki_lib_state_machine.vi"("State(s) in (\"\")"=w281) -> ("States Out"=w280:string)  [unwired: 14 in]
      }
      frame "Measure: Cryostat" {
        # "Your code here.\n(You can make a copy of, or modify, this frame)"
        n102 = Unbundle By Name(w286) -> ("Instruments.Magnet"=w291:refnum<class "Instrument.Cryostat.lvclass">, "Instruments.Temperature"=w290:refnum<class "Instrument.Cryostat.lvclass">)
        n103 = call-dynamic "Get Temperature.vi"("error in (no error)"=w289, "Instrument.Cryostat in"=w290) -> ("error out"=w292:errorcluster, "Temperature (K)"=w287:dbl)  [unwired: 6 in, 2 out]
        "Temp" <- w287
        n104 = call-dynamic "Get Magnet Field.vi"("error in (no error)"=w292, "Instrument.Cryostat in"=w291) -> ("error out"=w284:errorcluster, "B Field (T)"=w288:dbl)  [unwired: 6 in, 2 out]
        "Field (T)" <- w288
        n105 = Bundle By Name(cluster=w286, "Temperature"=w287, "Magnet"=w288) -> (w285:T8)
        n106 = call <vilib>:"Clear Errors.vi"("error in (no error)"=w284, "specific error code to clear (0: all)"=4000) -> ("error out"=w283:errorcluster)  [unwired: 4 in, 1 out]
        n107 = call <vilib>:"Add State(s) to Queue__jki_lib_state_machine.vi"("State(s) in (\"\")"=w294) -> ("States Out"=w293:string)  [unwired: 14 in]
      }
      frame "Measure: Lockin" {
        # "Your code here.\n(You can make a copy of, or modify, this frame)"
        n108 = Unbundle By Name(w298) -> ("Instruments.Lockin"=w306:refnum<class "Instrument.Lockin.lvclass">)
        n109 = call <userlib>:"waitForNewWaveforms.vi"("error in (no error)"=w308, "Instrument.Lockin in"=w306) -> ("error out"=w310:errorcluster, "Newest AI Waveform"=w296:waveform(dbl)[], "Instrument.Lockin out"=w311:refnum<class "Instrument.Lockin.lvclass">)  [unwired: 7 in]
        n110 = call <userlib>:"getAOconfig.vi"("error in (no error)"=w310, "Instrument.Lockin in"=w311) -> ("error out"=w309:errorcluster, "AOconfig"=w304:T6, "Instrument.Lockin out"=w312:refnum<class "Instrument.Lockin.lvclass">)  [unwired: 7 in]
        n111 = Index Array(array=w296) -> (element=w300:waveform(dbl))  [unwired: 1 in]
        n112 = call <userlib>:"getAO.vi"("error in (no error)"=w309, "Instrument.Lockin in"=w312) -> ("error out"=w307:errorcluster, "AO Waveforrm"=w305:waveform(dbl)[])  [unwired: 7 in, 1 out]
        n113 = Unbundle By Name(w300) -> ("Y"=w299:dbl[], "t0"=w301:timestamp, "dt"=w302:dbl)
        n114 = To Double Precision Float(number=w301) -> (double precision float=w303:dbl)
        n115 = for {
          tunnel: w302 -> [w318]
          tunnel: w303 -> [w316]
          tunnel: [w315] -> w295 mode=indexing
          tunnel: w299 -> [_] mode=indexing
          i -> [w319]
          n116 = Multiply(x=w319, y=w318) -> (x*y=w317:dbl)
          n117 = Add(x=w316, y=w317) -> (x+y=w315:dbl)
        }
        n118 = Bundle By Name(cluster=w298, "AI Waveform"=w296, "AOconfig"=w304, "AO Waveforrm"=w305, "time"=w295) -> (w297:T8)
        n119 = call <vilib>:"Add State(s) to Queue__jki_lib_state_machine.vi"("State(s) in (\"\")"=w314) -> ("States Out"=w313:string)  [unwired: 14 in]
      }
      frame "Measure: Filter and Decimate" {
        # "B"
        # "B"
        # "Template Separator\n(You can make a copy of, or modify, this frame)"
        n120 = Unbundle By Name(w323) -> ("time"=w328:dbl[], "AI Waveform"=w329:waveform(dbl)[])
        n121 = Unbundle By Name(w323) -> ("AO Waveforrm"=w327:waveform(dbl)[])
        n122 = for {
          tunnel: w329 -> [w352] mode=indexing
          tunnel: [w353] -> w332 mode=indexing
          tunnel: "offset" -> [w349] mode=indexing
          tunnel: "invert" -> [w351] mode=indexing
          n123 = Multiply(x=w352, y=w351) -> (x*y=w350:waveform(dbl))
          n124 = Add(x=w350, y=w349) -> (x+y=w353:waveform(dbl))
        }
        n125 = for {
          tunnel: "low cutoff freq: fl" -> [w338]
          tunnel: w327 -> [w342] mode=indexing
          tunnel: [w340] -> w324 mode=concatenating
          tunnel: "decimating factor" -> [w339]
          tunnel: "Enable Filter?" -> [w337]
          n126 = call "Decimate and Filter.vi"("Enabled?"=w337, "low cutoff freq: fl"=w338, "decimating factor"=w339, "Waveform in"=w342) -> ("Decimated and Filtered Array"=w341:dbl[])  [unwired: 6 in, 1 out]
          n127 = Build Cluster Array(w341) -> (w340:cluster{"Decimated and Filtered Array":dbl[]}[])
        }
        n128 = for {
          tunnel: "low cutoff freq: fl" -> [w344]
          tunnel: w332 -> [w348] mode=indexing
          tunnel: [w346] -> w325 mode=concatenating
          tunnel: "decimating factor" -> [w345]
          tunnel: "Enable Filter?" -> [w343]
          n129 = call "Decimate and Filter.vi"("Enabled?"=w343, "low cutoff freq: fl"=w344, "decimating factor"=w345, "Waveform in"=w348) -> ("Decimated and Filtered Array"=w347:dbl[])  [unwired: 6 in, 1 out]
          n130 = Build Cluster Array(w347) -> (w346:cluster{"Decimated and Filtered Array":dbl[]}[])
        }
        n131 = call "Decimate and Filter.vi"("Enabled?"="Enable Filter?", "low cutoff freq: fl"="low cutoff freq: fl", "decimating factor"="decimating factor", "Waveform in"=w328) -> ("Decimated and Filtered Array"=w326:dbl[])  [unwired: 6 in, 1 out]
        n132 = Bundle By Name(cluster=w323, "time (filtered)"=w326, "AI (filtered)"=w325, "AO (filtered)"=w324) -> (w322:T8)
        n133 = call <vilib>:"Add State(s) to Queue__jki_lib_state_machine.vi"("State(s) in (\"\")"=w336) -> ("States Out"=w335:string)  [unwired: 14 in]
      }
      frame "---------- File ----------" {
        # "Do not put any code in this frame.\n(It is a separator no-op. You can make a copy of this frame to create a new Macro frame)"
        n134 = call <vilib>:"Add State(s) to Queue__jki_lib_state_machine.vi"("State(s) in (\"\")"=w357) -> ("States Out"=w356:string)  [unwired: 14 in]
      }
      frame "File: Save" {
        # "Do not put any code in this frame.\n(It is a separator no-op. You can make a copy of this frame to create a new Macro frame)"
        n135 = Unbundle By Name(w371) -> ("Control Experiment"=w361:refnum<class "Control Experiment.lvclass">, "time (filtered)"=w370:dbl[], "Temperature"=w369:dbl, "Magnet"=w368:dbl, "AI (filtered)"=w365:cluster{"Decimated and Filtered Array":dbl[]}[], "AO (filtered)"=w363:cluster{"Decimated and Filtered Array":dbl[]}[])
        n136 = Build Array(w368) -> (w366:dbl[])
        n137 = Build Array(w369) -> (w367:dbl[])
        n138 = for {
          tunnel: w365 -> [_] mode=indexing
          tunnel: [w382] -> w364 mode=indexing
          i -> [w383]
          n139 = Increment(x=w383) -> (x+1=w386:i32)
          n140 = Number To Decimal String(number=w386) -> (decimal integer string=w384:string)  [unwired: 1 in]
          n141 = Concatenate Strings("AI" ("wavenames"), w384) -> (w382:string)
        }
        n142 = for {
          tunnel: [w377] -> w362 mode=indexing
          tunnel: w363 -> [_] mode=indexing
          i -> [w378]
          n143 = Increment(x=w378) -> (x+1=w381:i32)
          n144 = Number To Decimal String(number=w381) -> (decimal integer string=w379:string)  [unwired: 1 in]
          n145 = Concatenate Strings("AO" ("wavenames"), w379) -> (w377:string)
        }
        n146 = Build Cluster Array(w370, w367, w366) -> (w360:cluster{"time (filtered)":dbl[]}[])
        n147 = Build Array (concatenate)(w360, w365, w363) -> (w372:cluster{"Decimated and Filtered Array":dbl[]}[])
        n148 = Build Array (concatenate)(string[] ["time", "temp", "B"] ("wavenames (.Vx, etc)"), w364, w362) -> (w374:string[])
        n149 = call "Save Transport ITX File.vi"("error in (no error)"=w359, "Wavenames"=w374, "Data"=w372, "Control Experiment in"=w361) -> ("error out"=w358:errorcluster)  [unwired: 6 in, 1 out]
        n150 = call <vilib>:"Add State(s) to Queue__jki_lib_state_machine.vi"("State(s) in (\"\")"=w376) -> ("States Out"=w375:string)  [unwired: 14 in]
      }
    }
  }
  "error out" <- w1
  n151 = Unbundle By Name(w4) -> ("Transport"=→"Transport out":refnum<class "Transport.lvclass">)
